vi "getLocalVersions.vi"(8 "error in (no error)":errorcluster, 11 "hgHandler in":refnum<class "hgHandler.lvclass">) -> (0 "error out":errorcluster, 3 "hgHandler out":refnum<class "hgHandler.lvclass">, 4 "Local Versions":cluster{"version":string, "longHash":string}[](array[cluster]))   [LabVIEW 2013, in "hgHandler.lvclass"]
uses:
  hgHandler.lvclass
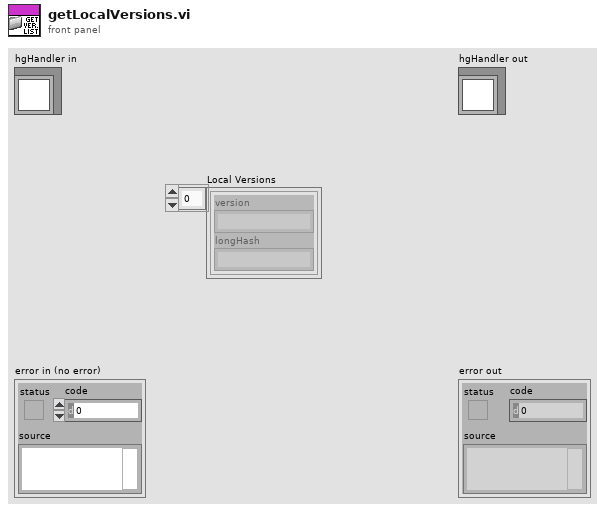
[diagram p1: front panel]
types:
  T1 = cluster{"standard output":string, "standard output":string}
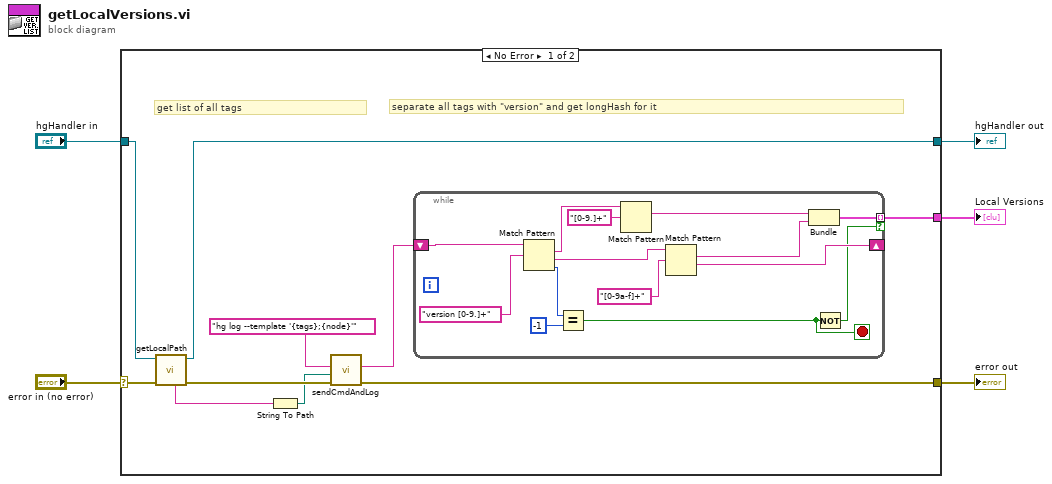
[diagram p0: block diagram]
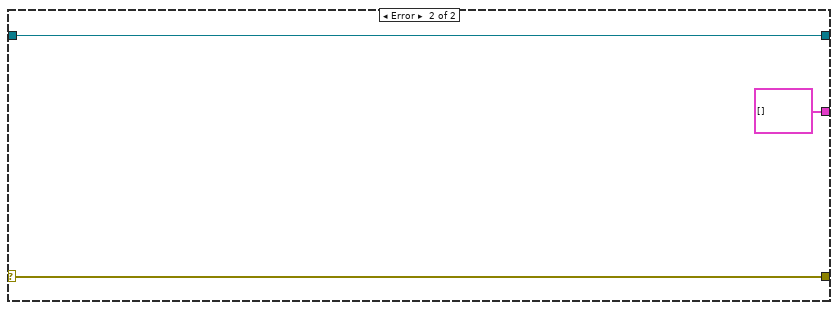
[diagram p2: hidden frame]
diagram:
  n1 = case shown="No Error" "error in (no error)" {
    selector: "error in (no error)" -> [w12 w32]
    tunnel: [w14 w32] -> w4
    tunnel: "hgHandler in" -> [w8 w31]
    tunnel: [w7 w31] -> w2
    tunnel: [w15 cluster{"Log":string, "Log":string}[] []] -> w1
    frame No Error {
      # "separate all tags with \"version\" and get longHash for it"
      # "get list of all tags"
      n2 = call-dynamic "getLocalPath.vi"("error in (no error)"=w12, "repoHandler in"=w8) -> ("error out"=w11:errorcluster, "repoHandler out"=w7:refnum<class "hgHandler.lvclass">, "Local Path"=w10:string)  [unwired: 7 in]
      n3 = String To Path(string=w10) -> (path=w9:path)
      n4 = call "sendCmdAndLog.vi"("error in (no error)"=w11, "working directory"=w9, "command"="hg log --template '{tags};{node}'" ("command line")) -> ("error out"=w14:errorcluster, "standard output"=w6:string)  [unwired: 6 in, 1 out]
      n5 = while {
        shift-right: [w23] -> _
        shift-left: w6 -> [w28]
        tunnel: [w21] -> w15 mode=indexing if=w19
        stop <- w25 stop-if-true
        n6 = Match Pattern(string=w28, regular expression="version [0-9.]+") -> (match substring=w18:string, after substring=w24:string, offset past match=w27:i32)  [unwired: 1 in, 1 out]
        n7 = Equal?(x=w27, y=-1) -> (x = y?=w25:bool)
        n8 = Match Pattern(string=w18, regular expression="[0-9.]+") -> (match substring=w16:string)  [unwired: 1 in, 3 out]
        n9 = Match Pattern(string=w24, regular expression="[0-9a-f]+") -> (match substring=w20:string, after substring=w23:string)  [unwired: 1 in, 2 out]
        n10 = Bundle("standard output"=w16, "standard output"=w20) -> (w21:T1)  [unwired: 1 in]
        n11 = Not(x=w25) -> (.not. x?=w19:bool)
      }
    }
    frame Error {
    }
  }
  "error out" <- w4
  "hgHandler out" <- w2
  "Local Versions" <- w1
